vi "读取Beverage.lvclass.vi"(8 "error in (no error)":errorcluster caption="错误输入（无错误）", 11 "Mocha输入":refnum<class "Mocha.lvclass">) -> (0 "error out":errorcluster caption="错误输出", 2 "Beverage.lvclass":refnum<class "Beverage.lvclass">, 3 "Mocha输出":refnum<class "Mocha.lvclass">)   [LabVIEW 2016, in "Mocha.lvclass"]
uses:
  Mocha.lvclass
  Beverage.lvclass
  Mocha.lvclass/Mocha.ctl
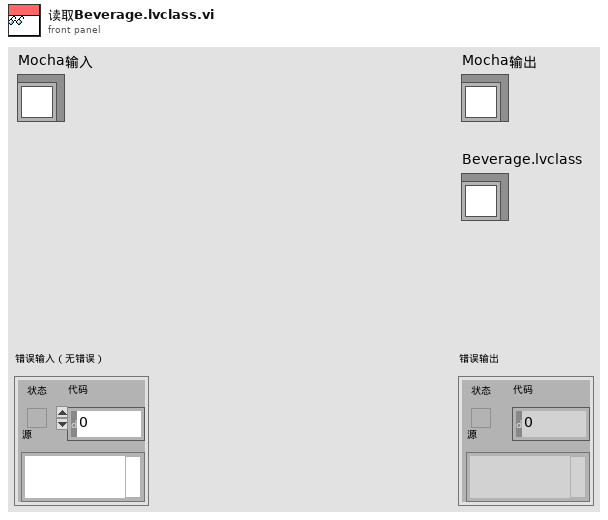
[diagram p1: front panel]
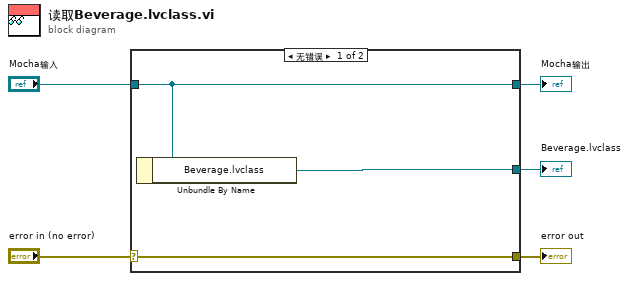
[diagram p0: block diagram]
diagram:
  n1 = case shown="无错误" "error in (no error)" {
    selector: "error in (no error)" -> [w8 w9]
    tunnel: [w8 w9] -> w4
    tunnel: [w7 w10] -> w2
    tunnel: "Mocha输入" -> [w7 w10]
    tunnel: [w6 _] -> w1
    frame No Error {
      n2 = Unbundle By Name(w7) -> ("Beverage.lvclass"=w6:refnum<class "Beverage.lvclass">)
    }
    frame Error {
    }
  }
  "error out" <- w4
  "Mocha输出" <- w2
  "Beverage.lvclass" <- w1
